vi "SNA Convert Frequency to MHz.vi"(10 "Units":enum16{"Hz", "kHz", "MHz", "GHz"}(ring)=enum."MHz", 11 "Frequency":dbl) -> (3 "Converted Frequency":dbl)   [LabVIEW 2011]
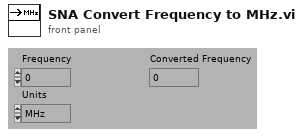
[diagram p1: front panel]
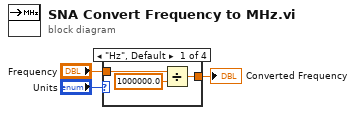
[diagram p0: block diagram]
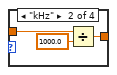
[diagram p2: hidden frame]
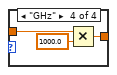
[diagram p4: hidden frame]
diagram:
  n1 = case shown="\"Hz\", Default" "Units" {
    tunnel: "Frequency" -> [w6 w8 w10 w13]
    tunnel: [w5 w7 w10 w12] -> w1
    frame "Hz", Default {
      n2 = Divide(x=w6, y=1000000.0) -> (x/y=w5:dbl)
    }
    frame "kHz" {
      n3 = Divide(x=w8, y=1000.0) -> (x/y=w7:dbl)
    }
    frame "MHz" {
    }
    frame "GHz" {
      n4 = Multiply(x=w13, y=1000.0) -> (x*y=w12:dbl)
    }
  }
  "Converted Frequency" <- w1
